vi "roboRIO v1.0 Unreserve I2C.vi"(7 "Allow multiple opens?":bool, 8 "error in (no error)":errorcluster, 10 "I2C Channel":T2, 11 "myRIO FPGA Ref Out":T1) -> (0 "error out":errorcluster)   [LabVIEW 2021]
uses:
  <vilib>/myRIO/Common/Instrument Driver Framework/myRIO v1.0/I2C/typedefs/I2C Channels Enum.ctl
  <vilib>/myRIO/Common/Instrument Driver Framework/Utilities/typedefs/Generic FPGA Reference.ctl
  <vilib>/myRIO/Common/Instrument Driver Framework/roboRIO v1.0/Resource Manager/vis/roboRIO v1.0 Unreserve Channel.vi
  <vilib>/myRIO/Common/Instrument Driver Framework/roboRIO v1.0/Resource Manager/vis/roboRIO v1.0 Create Configuration List.vi
  <vilib>/myRIO/Common/Instrument Driver Framework/roboRIO v1.0/Resource Manager/vis/roboRIO v1.0 Build Mutex Name.vi
  <vilib>/myRIO/Common/Instrument Driver Framework/Utilities/vis/Configuration Manager.vi
  <vilib>/myRIO/Common/Instrument Driver Framework/Utilities/vis/IO Manager.vi
  <vilib>/Utility/error.llb/Error Cluster From Error Code.vi
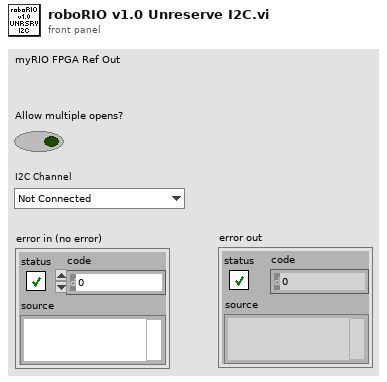
[diagram p1: front panel]
types:
  T1 = typedef "Generic FPGA Reference.ctl" = refnum<k20>
  T2 = typedef "I2C Channels Enum.ctl" = enum16{"Not Connected", "A/I2C", "B/I2C", "I2C/I2C"}
  T3 = typedef "roboRIO v1.0 Channel Reservation List.ctl" = T4[]
  T4 = typedef "roboRIO v1.0 Channel Reservation Info.ctl" = cluster{"Channel Name":string, "Connector":T5, "Mutex ID":i32}
  T5 = typedef "roboRIO v1.0 Connector List.ctl" = enum32{"None", "ConnectorB", "ConnectorI2C", "ConnectorDIO", "ConnectorRSL", "ConnectorRELAY", "ConnectorAI", "ConnectorPWM", "ConnectorSPI"}
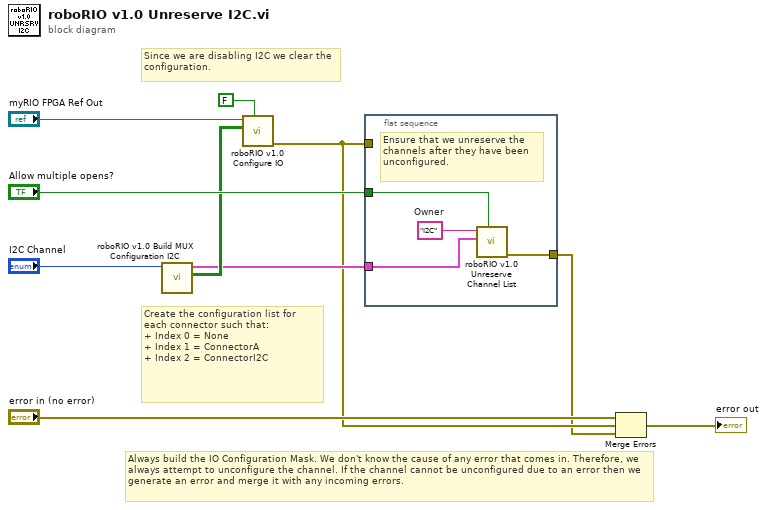
[diagram p0: block diagram]
diagram:
  # "Since we are disabling I2C we clear the configuration."
  # "Always build the IO Configuration Mask. We don't know the cause of any error that comes in. Therefore, we always attempt to unconfigure the channel. If the channel cannot be unconfigured due to an error then we generate an error and merge it with any incoming errors."
  # "Create the configuration list for each connector such that:\n+ Index 0 = None\n+ Index 1 = ConnectorA\n+ Index 2 = ConnectorI2C"
  n1 = call <vilib>:"roboRIO v1.0 Build MUX Configuration I2C.vi"("Channel"="I2C Channel") -> ("Configuration Bitmask Array"=w4:bool[][], "Channel Reservation List"=w3:T3)  [unwired: 9 in]
  n2 = call <vilib>:"roboRIO v1.0 Configure IO.vi"("Value"=FALSE ("Clear?"), "Bitmask Array"=w4, "myRIO FPGA Ref In"="myRIO FPGA Ref Out") -> ("error out"=w2:errorcluster)  [unwired: 8 in]
  n3 = flat-sequence {
    tunnel: "Allow multiple opens?" -> [w14]
    tunnel: w3 -> [w12]
    tunnel: w2 -> [_]
    tunnel: [w11] -> w1
    frame #0 {
      w13 = "I2C"  # Owner
      # "Ensure that we unreserve the channels after they have been unconfigured."
      n4 = call <vilib>:"roboRIO v1.0 Unreserve Channel List.vi"("Allow multiple opens?"=w14, "Channel Reservation List"=w12, "Owner"=w13) -> ("error out"=w11:errorcluster)  [unwired: 8 in]
    }
  }
  n5 = Merge Errors("error in (no error)", w2, w1) -> (→"error out":errorcluster)
